vi "End Effector Motors TestCode.vi"() -> ()   [LabVIEW 2014]
panel:
  in  "Foam Gnome Motor Control":dbl(slide) scale=-1.0..1.0
  in  "End Effector Motor Control 2":dbl(slide) scale=-1.0..1.0
  in  "End Effector Motor Control 1":dbl(slide) scale=-1.0..1.0
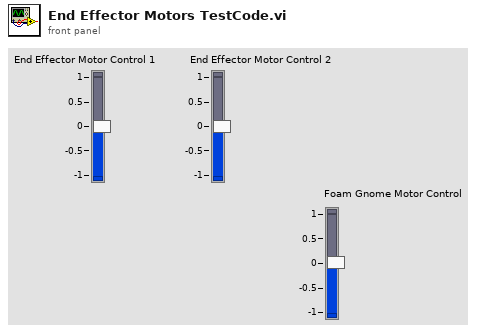
[diagram p1: front panel]
types:
  T1 = typedef "WPI_MotorControlDeviceRef.ctl" = cluster{"DeviceStatus":errorcluster, "Type":T2, "PWM":cluster{"Controller":T3, "PWM Channel":T4, "DeadBand":T5}, "CAN":cluster{"Device Number":u8, "Control Mode":T6, "Semaphore":T7, "Max Vout":dbl, "TalonSRX Control Mode":T8}, "Invert":bool, "TransformRef":T9, "InvTransformRef":T9}
  T2 = typedef "WPI_MotorControlType.ctl" = enum16{"PWM", "CAN", "CANTalonSRX"}
  T3 = typedef "FPGA_TypedefDigitalModule.ctl" = enum16{"Controller 1"}
  T4 = typedef "FPGA_DIOPWMChannel.ctl" = enum8{"PWM 0", "PWM 1", "PWM 2", "PWM 3", "PWM 4", "PWM 5", "PWM 6", "PWM 7", "PWM 8", "PWM 9", "PWM MXP 0", "PWM MXP 1", "PWM MXP 2", "PWM MXP 3", "PWM MXP 4", "PWM MXP 5", "PWM MXP 6", "PWM MXP 7", "PWM MXP 8", "PWM MXP 9", "Invalid"}
  T5 = typedef "WPI_PWMDeadband.ctl" = cluster{"Name":string, "maxPositivePwm":i32, "minPositivePwm":i32, "centerPwm":i32, "maxNegativePwm":i32, "minNegativePwm":i32, "angularRange":u16}
  T6 = typedef "WPI_CANJaguar_ControlMode.ctl" = enum8{"Percent VBus", "Current", "Speed", "Position", "Voltage"}
  T7 = typedef "Semaphore RefNum" = refnum<k1>
  T8 = typedef "WPI_CANTalonSRX_APIControlMode.ctl" = enum8{"Percent VBus", "Speed", "Position", "Slave", "Unchanged / Invalid"}
  T9 = typedef "WPI_PWMTransform_ConPane.ctl" = refnum<vi>
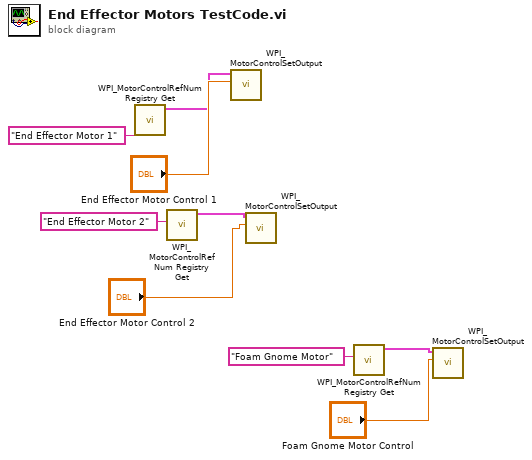
[diagram p0: block diagram]
diagram:
  n1 = call <vilib>:"WPI_MotorControlRefNum Registry Get.vi"("refnum name"="End Effector Motor 1") -> ("MotorControlDevRef"=w4:T1)  [unwired: 9 in, 1 out]
  n2 = call <vilib>:"WPI_MotorControlRefNum Registry Get.vi"("refnum name"="End Effector Motor 2") -> ("MotorControlDevRef"=w5:T1)  [unwired: 9 in, 1 out]
  n3 = call <vilib>:"WPI_MotorControlSetOutput.vi"("Output"="End Effector Motor Control 1", "MotorControlDevRef"=w4) -> ()  [unwired: 7 in, 3 out]
  n4 = call <vilib>:"WPI_MotorControlSetOutput.vi"("Output"="End Effector Motor Control 2", "MotorControlDevRef"=w5) -> ()  [unwired: 7 in, 3 out]
  n5 = call <vilib>:"WPI_MotorControlRefNum Registry Get.vi"("refnum name"="Foam Gnome Motor") -> ("MotorControlDevRef"=w2:T1)  [unwired: 9 in, 1 out]
  n6 = call <vilib>:"WPI_MotorControlSetOutput.vi"("Output"="Foam Gnome Motor Control", "MotorControlDevRef"=w2) -> ()  [unwired: 7 in, 3 out]
